vi "実測定画面.vi"(4 "測定値MAX/MIN":string[][](table), 7 "実測設定項目配列_\nメインからの転記":T1[](array[typedef]) {"測定モード" items=["単発測定モード", "連続測定モード", "多点測定モード"]}, 11 "測定周期/ms_制御器":dbl) -> (8 "実測設定項目配列_\nゲージIOへ転記用":T1[](array[typedef]) {"測定モード" items=["単発測定モード", "連続測定モード", "多点測定モード"]}, 10 "実測設定項目配列_\n多点測定メイン転記用":T1[](array[typedef]) {"測定モード" items=["単発測定モード", "連続測定モード", "多点測定モード"]}, 15 "測定周期/ms_表示器":dbl)   [LabVIEW 2021]
panel:
  out "文字列":string
  out "実測値MAXエラー判定 4":bool
  out "実測値MAXエラー判定 3":bool
  out "実測値MAXエラー判定 2":bool
  out "実測値MAXエラー判定":bool
  out "測定値MAX/MIN_グローバルから転記":string[][](table)
  in  "測定値MAX/MINリセット用 2":string[][](table)
  in  "測定値MAX/MIN_多点測定":string[][](table)
  in  "測定値MAX/MINリセット用":string[][](table)
  in  "実測ONOFFボタン":T2
  out "実測値":string[][](table)
  # "実測定画面"
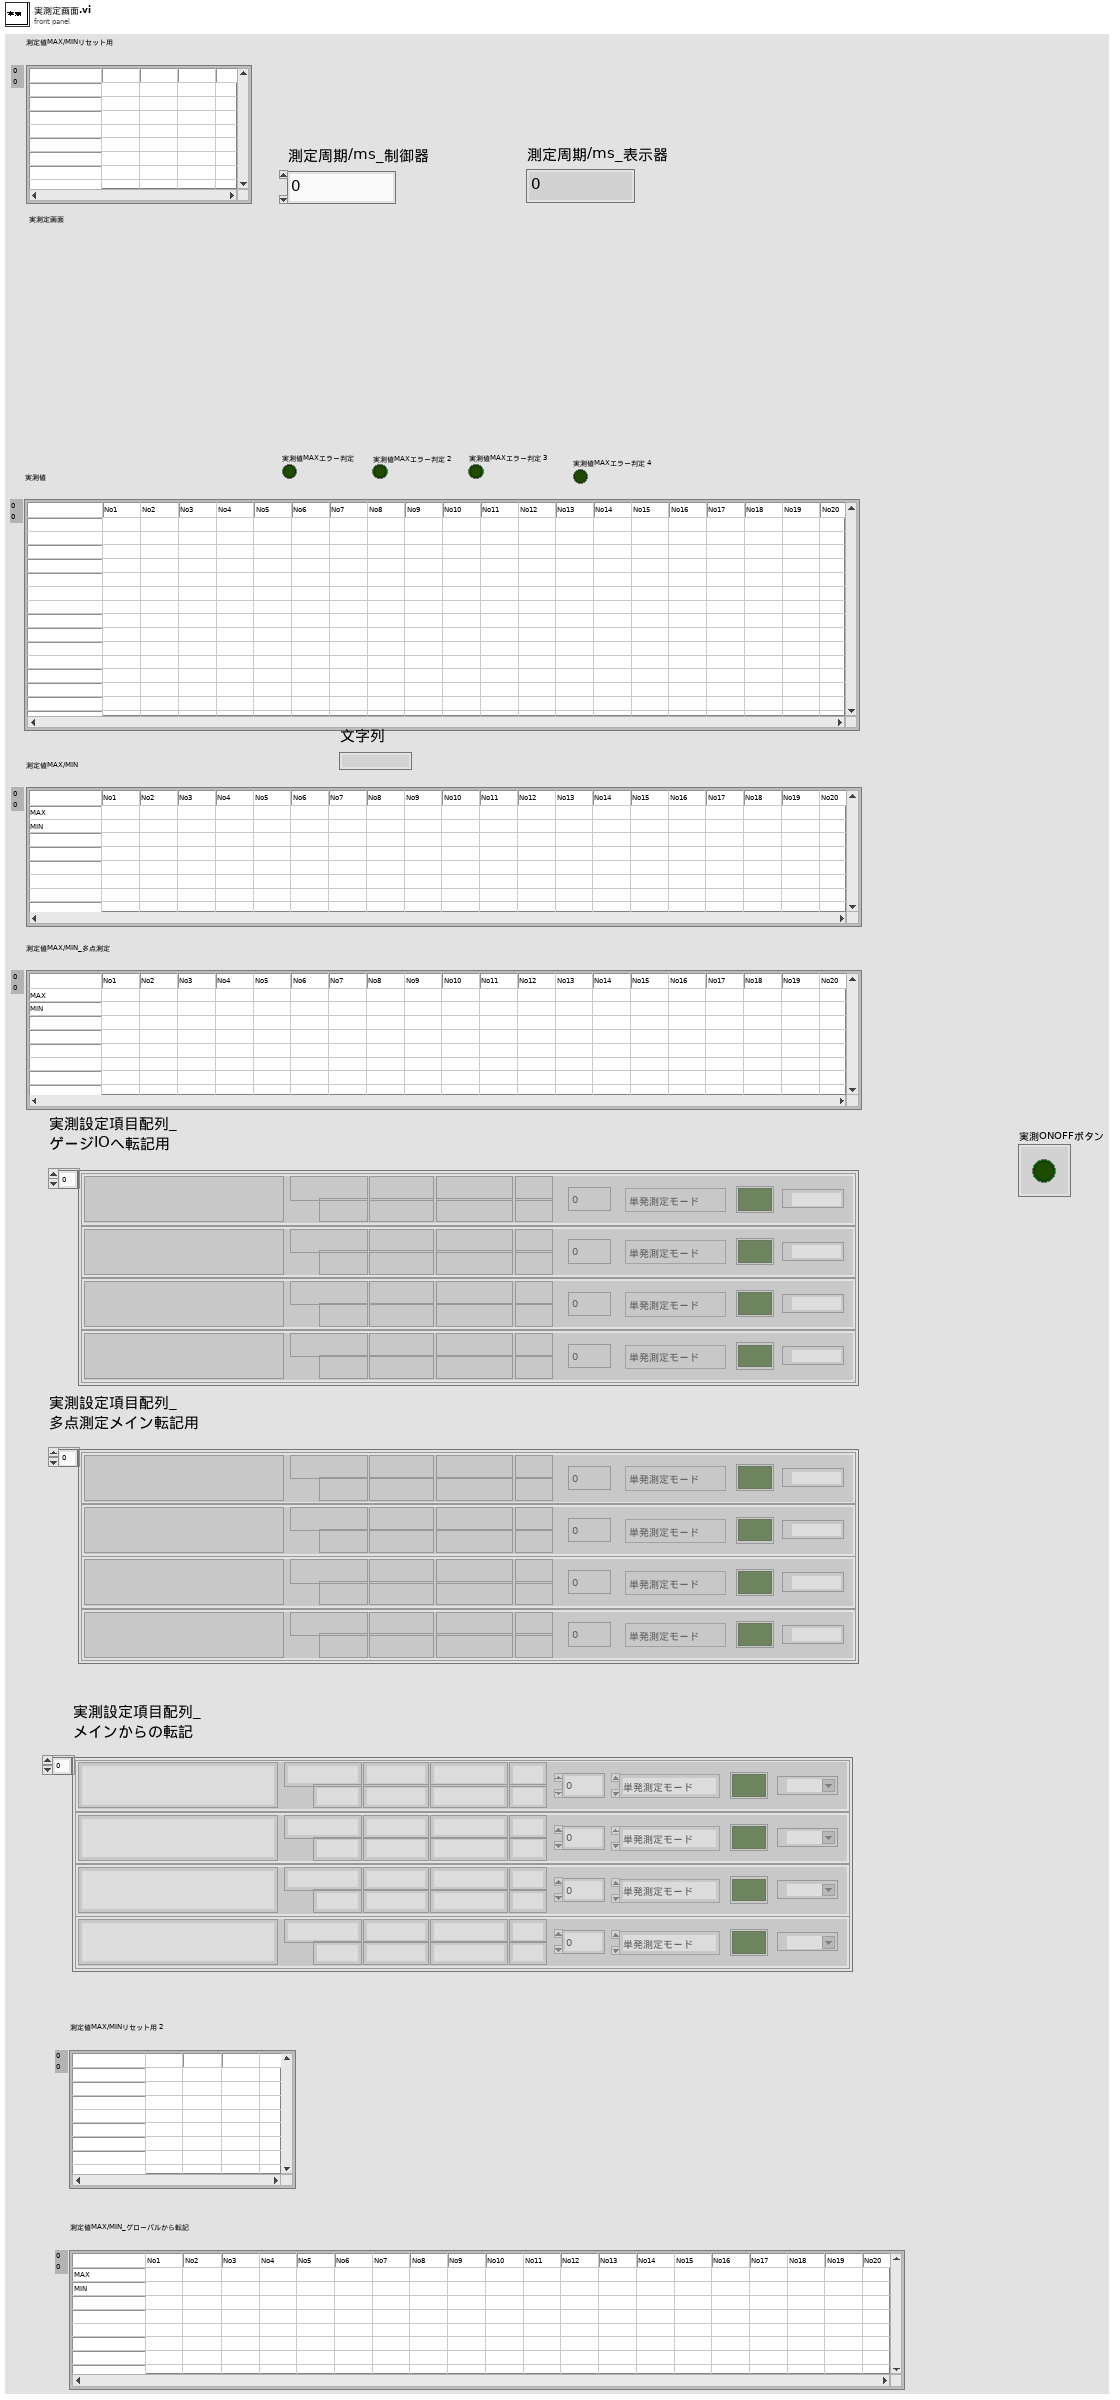
[diagram p1: front panel]
types:
  T1 = typedef "設定全項目制御器.ctl" = cluster{"規格":string, "規格上限":string, "規格下限":string, "ポートNo.":dbl, "測定モード":u16, "規格単位":string, "品質チェック項目":string, "測定周期":dbl, "実測値MAX":string, "実測値MIN":string, "実測値(MAX)":string, "実測値(MIN)":string, "測定画面表示ボタン":bool, "ゲージポートNo":refnum<visa-resource-name>}
  T2 = typedef "ONOFFボタン制御器.ctl" = cluster{"使用ON/OFF":bool}
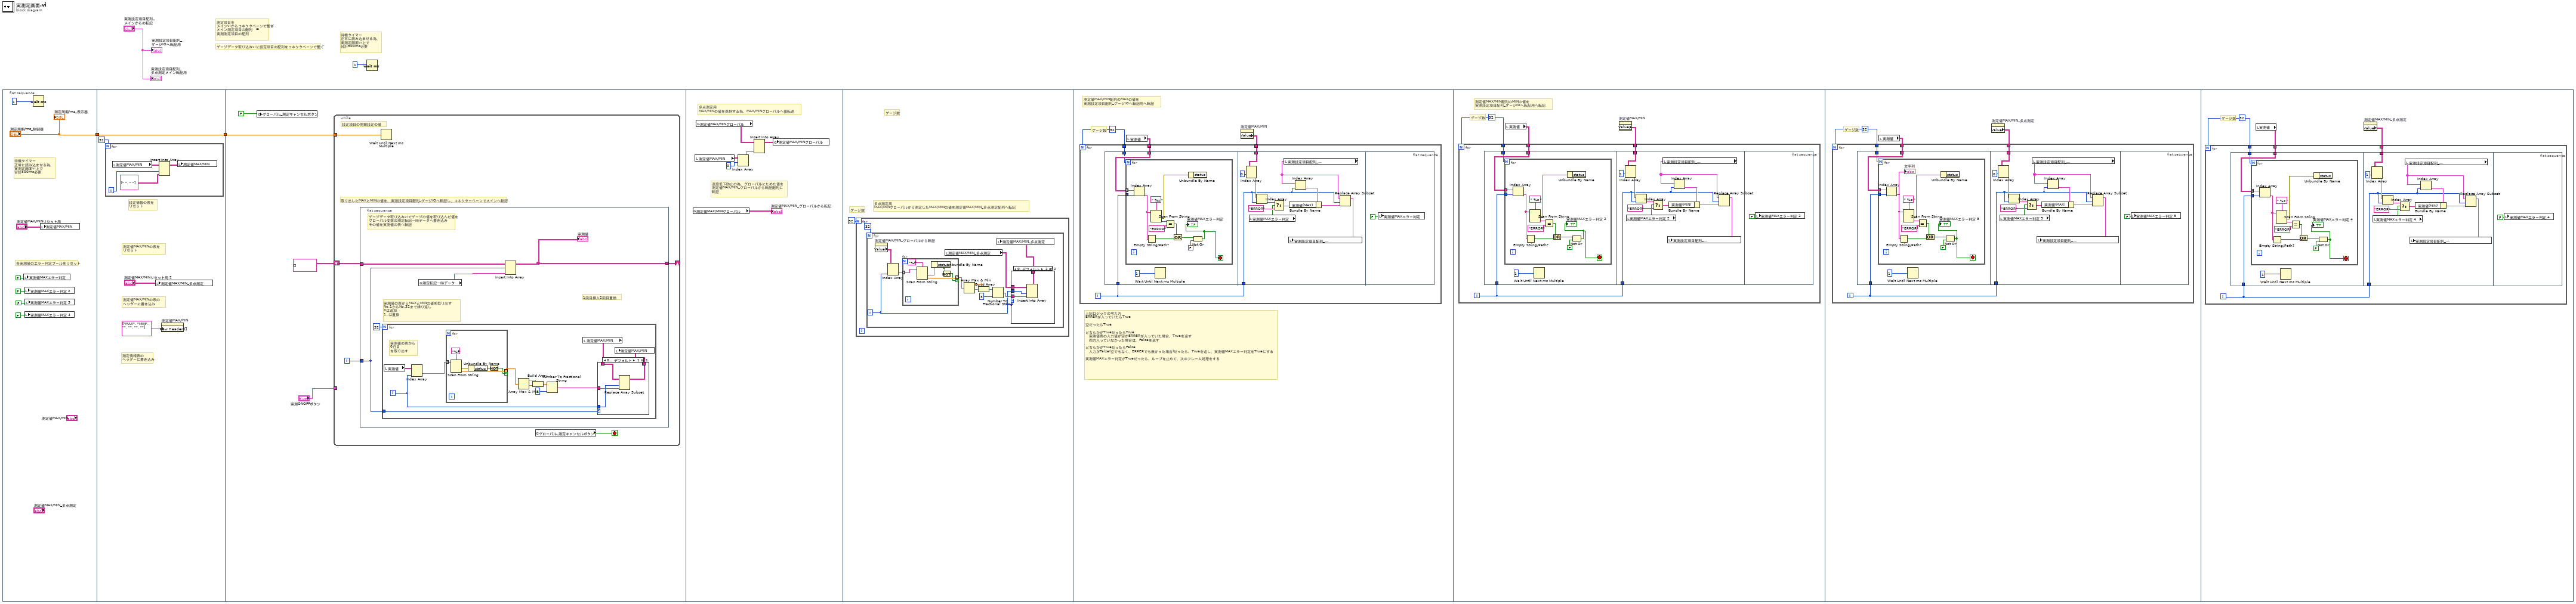
[diagram p0: block diagram]
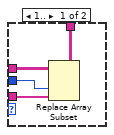
[diagram p2: hidden frame]
diagram:
  # "測定項目を\nメインviからコネクタペーンで繋ぎ\nメイン測定項目の配列　=\n実測測定項目の配列"
  # "ゲージデータ取り込みviに設定項目の配列をコネクタペーンで繋ぐ"
  # "待機タイマー\n正常に読み込ませる為、\n実測定画面vi上で\n合計500ms必要"
  n1 = flat-sequence {
    tunnel: ["測定周期/ms_制御器"] -> w4
    tunnel: w4 -> [w14]
    tunnel: [w14] -> w3
    tunnel: w3 -> [w21]
    frame #0 {
      # "各実測値のエラー判定ブールをリセット"
      # "待機タイマー\n正常に読み込ませる為、\n実測定画面vi上で\n合計500ms必要"
      n2 = local write "実測値MAXエラー判定"(FALSE) -> ()
      n3 = local write "実測値MAXエラー判定 2"(FALSE) -> ()
      n4 = local write "実測値MAXエラー判定 4"(FALSE) -> ()
      n5 = local write "実測値MAXエラー判定 3"(FALSE) -> ()
      n6 = Wait (ms)(milliseconds to wait=1) -> ()  [unwired: 1 out]
      n7 = local write "測定値MAX/MIN"("測定値MAX/MINリセット用") -> ()
      "測定周期/ms_表示器" <- "測定周期/ms_制御器"
    }
    frame #1 {
      # "測定情報表の\nヘッダーに書き込み"
      # "測定値MAX/MINの表の\nヘッダーに書き込み"
      # "測定値MAX/MINの表を\nリセット"
      # "設定情報の表を\nリセット"
      n8 = for {
        N: 32 -> [_]
        i -> [w16]
        n9 = local read "測定値MAX/MIN"() -> (w19:string[][])
        n10 = Insert Into Array(array=w19, index (col)=w16, new element=string[][] [[" "], [" "]]) -> (w18:string[][])  [unwired: 1 in]
        n11 = local write "測定値MAX/MIN"(w18) -> ()
      }
      n12 = local write "測定値MAX/MIN_多点測定"("測定値MAX/MINリセット用 2") -> ()
      n13 = property on="測定値MAX/MIN" class="Tbl (指定)"("Row Headers[]"=string[] ["MAX", "MIN", "", "", "", ""]) -> ()  [unwired: 2 in, 2 out]
    }
    frame #2 {
      n14 = global write "測定キャンセルボタン.vi" "グローバル_測定キャンセルボタン"(FALSE) -> ()
      n15 = while "Whileループ" {
        tunnel: "実測ONOFFボタン" -> [_]
        shift-right: [w26] -> _
        shift-left: string[][] [] ("配列") -> [w28]
        tunnel: w21 -> [w24]
        i -> [w27]
        stop <- w25 stop-if-true
        # "取り出したMAXとMINの値を、実測設定項目配列_ゲージIOへ転記し、コネクターペーンでメインへ転記"
        # "設定項目の周期設定の値"
        n16 = flat-sequence {
          tunnel: w28 -> [w33]
          tunnel: w27 -> [w29]
          tunnel: [w32] -> w26
          frame #0 {
            # "1回目挿入2回目置換"
            # "実測値の表からMAXとMINの値を取り出す\nNo.1からNo.32まで繰り返し\n0は追加\n1..は置換"
            # "ゲージデータ取り込みviでゲージの値を取り込んだ値を\nグローバル変数の測定転記一時データへ書き込み\nその値を実測値の表へ転記"
            n17 = for {
              N: 32 -> [_]
              tunnel: w29 -> [w41]
              i -> [w37]
              # "実測値の表から\n0行目\nを取り出す"
              n18 = local read "実測値"() -> (w45:string[][])
              n19 = Index Array(array=w45, index (col)=w37) -> (element=w34:string[])  [unwired: 1 in]
              n20 = for {
                tunnel: w34 -> [w54] mode=indexing
                tunnel: [w53] -> w42 mode=indexing if=w50
                n21 = Scan From String(format string="%f" ("形式文字列"), input string=w54) -> (error out=w52:errorcluster, output 1=w53:dbl)  [unwired: 3 in, 2 out]
                n22 = Unbundle By Name(w52) -> ("status"=w51:bool)
                n23 = Not(x=w51) -> (.not. x?=w50:bool)
              }
              n24 = Array Max & Min(array=w42) -> (max value=w36:dbl, min value=w44:dbl)  [unwired: 2 out]
              n25 = Build Array(w36, w44) -> (w43:dbl[])
              n26 = Number To Fractional String(number=w43, precision (6)=3) -> (F-format string=w35:string[])  [unwired: 2 in]
              n27 = local read "測定値MAX/MIN"() -> (w40:string[][])
              n28 = case shown="0.., デフォルト" w41 {
                tunnel: [w48] -> w39
                tunnel: w40 -> [w49]
                tunnel: w37 -> [w47]
                tunnel: w35 -> [w46]
                frame 0.., Default {
                  n29 = Replace Array Subset(array=w49, new element=w46, index (col)=w47) -> (w48:string[][])  [unwired: 1 in]
                }
              }
              n30 = local write "測定値MAX/MIN"(w39) -> ()
            }
            n31 = global read "測定データ転記.vi" "測定転記一時データ"() -> (w31:string[])
            n32 = Insert Into Array(array=w33, index (row)=w29, new element=w31) -> (w32:string[][])  [unwired: 1 in]
            "実測値" <- w32
          }
        }
        n33 = Wait Until Next ms Multiple(millisecond multiple=w24) -> ()  [unwired: 1 out]
        n34 = global read "測定キャンセルボタン.vi" "グローバル_測定キャンセルボタン"() -> (w25:bool)
      }
    }
    frame #3 {
      # "速度低下防止の為、グローバルにためた値を\n測定値MAX/MIN_グローバルから転記配列に\n転記"
      # "多点測定用\nMAX/MINの値を保持する為、MAX/MINグローバルへ値転送"
      n35 = global read "測定値MAXMIN_G.vi" "測定値MAX/MINグローバル"() -> (→"測定値MAX/MIN_グローバルから転記":string[][])
      n36 = local read "測定値MAX/MIN"() -> (w58:string[][])
      n37 = global read "測定値MAXMIN_G.vi" "測定値MAX/MINグローバル"() -> (w61:string[][])
      n38 = Index Array(array=w58, index (row)=0) -> (element=w59:string[])  [unwired: 1 in]
      n39 = Insert Into Array(array=w61, new element=w59) -> (w60:string[][])  [unwired: 2 in]
      n40 = global write "測定値MAXMIN_G.vi" "測定値MAX/MINグローバル"(w60) -> ()
    }
    frame #4 {
      # "多点測定用\nMAX/MINグローバルから測定したMAX/MINの値を測定値MAX/MIN_多点測定配列へ転記"
      # "ゲージ数"
      # "ゲージ数"
      n41 = for {
        N: 32 -> [_]
        n42 = for {
          N: 32 -> [_]
          i -> [w67]
          n43 = property on="測定値MAX/MIN_グローバルから転記" class="Tbl (指定)"() -> ("Value"=w65:string[][])  [unwired: 2 in, 2 out]
          n44 = Index Array(array=w65, index (col)=w67) -> (element=w71:string[])  [unwired: 1 in]
          n45 = for {
            tunnel: w71 -> [w88] mode=indexing
            tunnel: [w86] -> w70 mode=indexing if=w84
            n46 = Scan From String(format string="%f" ("形式文字列"), input string=w88) -> (error out=w85:errorcluster, output 1=w86:dbl)  [unwired: 3 in, 2 out]
            n47 = Unbundle By Name(w85) -> ("status"=w83:bool)
            n48 = Not(x=w83) -> (.not. x?=w84:bool)
          }
          n49 = local read "測定値MAX/MIN_多点測定"() -> (w69:string[][])
          n50 = Array Max & Min(array=w70) -> (max value=w74:dbl, min value=w66:dbl)  [unwired: 2 out]
          n51 = Build Array(w74, w66) -> (w73:dbl[])
          n52 = Number To Fractional String(number=w73, precision (6)=3) -> (F-format string=w72:string[])  [unwired: 2 in]
          n53 = case shown="0, デフォルト" w67 {
            tunnel: [w77 w80] -> w68
            tunnel: w69 -> [w78 w82]
            tunnel: w67 -> [w75 w79]
            tunnel: w72 -> [w76 w81]
            frame 1.. {
              n54 = Replace Array Subset(array=w78, new element=w76, index (col)=w75) -> (w77:string[][])  [unwired: 1 in]
            }
            frame 0, Default {
              n55 = Insert Into Array(array=w82, index (col)=w79, new element=w81) -> (w80:string[][])  [unwired: 1 in]
            }
          }
          n56 = local write "測定値MAX/MIN_多点測定"(w68) -> ()
        }
      }
    }
    frame #5 {
      w90 = 32
      # "上記ロジックの考え方\nERRERが入っていたらTrue\n\n空だったらTrue\n\nどちらかがTrueだったらTrue\n　実測値表の入力値が空かERRERが入っていた場合、Trueを返す\n　両方入っていなかった場合は、Falseを返す　\n\nどちらかがTrueだったらFalse\n　入力がFalse(空でもなく、ERRERでも無かった場合)だったら、Trueを返し、実測値MAXエラー判定をTrueにする\n\n実測値MAXエラー判定がTrueだったら、ループを止めて、次のフレーム処理をする"
      # "測定値MAX/MIN配列のMAXの値を\n実測設定項目配列_ゲージIOへ転記用へ転記"
      # "ゲージ数"
      n57 = local read "実測値"() -> (w91:string[][])
      n58 = property on="測定値MAX/MIN" class="Tbl (指定)"() -> ("Value"=w89:string[][])  [unwired: 2 in, 2 out]
      n59 = for {
        N: w90 -> [_]
        tunnel: w91 -> [w95]
        tunnel: w89 -> [w94]
        tunnel: w90 -> [w93]
        i -> [w92]
        n60 = flat-sequence {
          tunnel: w95 -> [w98]
          tunnel: w93 -> [w97]
          tunnel: w92 -> [w96]
          tunnel: w94 -> [w113]
          tunnel: w92 -> [w112]
          frame #0 {
            n61 = for {
              N: w97 -> [_]
              tunnel: w98 -> [w104] mode=indexing
              tunnel: w96 -> [w101]
              stop <- w100 stop-if-true
              n62 = Index Array(array=w104, index=w101) -> (element=w103:string)
              n63 = Empty String/Path?(string/path=w103) -> (empty?=w102:bool)
              n64 = Scan From String(format string=" %s " ("形式文字列"), input string=w103) -> (error out=w110:errorcluster, output 1=w109:string)  [unwired: 3 in, 2 out]
              n65 = Equal?(x=w109, y="ERROR") -> (x = y?=w107:bool)
              n66 = Or(x=w107, y=w102) -> (x .or. y?=w105:bool)
              n67 = Unbundle By Name(w110) -> ()  [unwired: 1 out]
              n68 = Not Or(1:FALSE, 2:w105) -> (0:w100:bool)
              "実測値MAXエラー判定" <- w100
            }
            n69 = Wait Until Next ms Multiple(millisecond multiple=u32 1 ("ミリ秒倍数")) -> ()  [unwired: 1 out]
          }
          frame #1 {
            n70 = Index Array(array=w113, index (row)=0) -> (element=w119:string[])  [unwired: 1 in]
            n71 = local read "実測値MAXエラー判定"() -> (w120:bool)
            n72 = Index Array(array=w119, index=w112) -> (element=w123:string)
            n73 = Select(t=w123, s=w120, f="ERROR") -> (s? t:f=w121:string)
            n74 = local read "実測設定項目配列_\nゲージIOへ転記用"() -> (w117:T1[])
            n75 = Index Array(array=w117, index=w112) -> (element=w114:T1)
            n76 = Bundle By Name(cluster=w114, "実測値(MAX)"=w121) -> (w115:T1)
            n77 = Replace Array Subset(array=w117, new element=w115, index=w112) -> (w116:T1[])
            n78 = local write "実測設定項目配列_\nゲージIOへ転記用"(w116) -> ()
          }
          frame #2 {
            n79 = local write "実測値MAXエラー判定"(FALSE) -> ()
          }
        }
      }
    }
    frame #6 {
      w127 = 32
      # "ゲージ数"
      # "測定値MAX/MIN配列のMINの値を\n実測設定項目配列_ゲージIOへ転記用へ転記"
      n80 = local read "実測値"() -> (w126:string[][])
      n81 = property on="測定値MAX/MIN" class="Tbl (指定)"() -> ("Value"=w125:string[][])  [unwired: 2 in, 2 out]
      n82 = for {
        N: w127 -> [_]
        tunnel: w126 -> [w131]
        tunnel: w125 -> [w130]
        tunnel: w127 -> [w129]
        i -> [w128]
        n83 = flat-sequence {
          tunnel: w131 -> [w134]
          tunnel: w129 -> [w133]
          tunnel: w128 -> [w132]
          tunnel: w130 -> [w149]
          tunnel: w128 -> [w148]
          frame #0 {
            n84 = for {
              N: w133 -> [_]
              tunnel: w134 -> [w140] mode=indexing
              tunnel: w132 -> [w137]
              stop <- w136 stop-if-true
              n85 = Index Array(array=w140, index=w137) -> (element=w139:string)
              n86 = Empty String/Path?(string/path=w139) -> (empty?=w138:bool)
              n87 = Scan From String(format string=" %s " ("形式文字列"), input string=w139) -> (error out=w146:errorcluster, output 1=w145:string)  [unwired: 3 in, 2 out]
              n88 = Equal?(x=w145, y="ERROR") -> (x = y?=w143:bool)
              n89 = Or(x=w143, y=w138) -> (x .or. y?=w141:bool)
              n90 = Unbundle By Name(w146) -> ()  [unwired: 1 out]
              n91 = Not Or(1:FALSE, 2:w141) -> (0:w136:bool)
              "実測値MAXエラー判定 2" <- w136
            }
            n92 = Wait Until Next ms Multiple(millisecond multiple=u32 1 ("ミリ秒倍数")) -> ()  [unwired: 1 out]
          }
          frame #1 {
            n93 = Index Array(array=w149, index (row)=1) -> (element=w155:string[])  [unwired: 1 in]
            n94 = local read "実測値MAXエラー判定 2"() -> (w156:bool)
            n95 = Index Array(array=w155, index=w148) -> (element=w159:string)
            n96 = Select(t=w159, s=w156, f="ERROR") -> (s? t:f=w157:string)
            n97 = local read "実測設定項目配列_\nゲージIOへ転記用"() -> (w153:T1[])
            n98 = Index Array(array=w153, index=w148) -> (element=w150:T1)
            n99 = Bundle By Name(cluster=w150, "実測値(MIN)"=w157) -> (w151:T1)
            n100 = Replace Array Subset(array=w153, new element=w151, index=w148) -> (w152:T1[])
            n101 = local write "実測設定項目配列_\nゲージIOへ転記用"(w152) -> ()
          }
          frame #2 {
            n102 = local write "実測値MAXエラー判定 2"(FALSE) -> ()
          }
        }
      }
    }
    frame #7 {
      w163 = 32
      # "ゲージ数"
      n103 = local read "実測値"() -> (w162:string[][])
      n104 = property on="測定値MAX/MIN_多点測定" class="Tbl (指定)"() -> ("Value"=w161:string[][])  [unwired: 2 in, 2 out]
      n105 = for {
        N: w163 -> [_]
        tunnel: w162 -> [w167]
        tunnel: w161 -> [w166]
        tunnel: w163 -> [w165]
        i -> [w164]
        n106 = flat-sequence {
          tunnel: w167 -> [w170]
          tunnel: w165 -> [w169]
          tunnel: w164 -> [w168]
          tunnel: w166 -> [w185]
          tunnel: w164 -> [w184]
          frame #0 {
            n107 = for {
              N: w169 -> [_]
              tunnel: w170 -> [w176] mode=indexing
              tunnel: w168 -> [w174]
              stop <- w172 stop-if-true
              n108 = Index Array(array=w176, index=w174) -> (element=w173:string)
              "文字列" <- w173
              n109 = Empty String/Path?(string/path=w173) -> (empty?=w175:bool)
              n110 = Scan From String(format string=" %s " ("形式文字列"), input string=w173) -> (error out=w182:errorcluster, output 1=w181:string)  [unwired: 3 in, 2 out]
              n111 = Equal?(x=w181, y="ERROR") -> (x = y?=w179:bool)
              n112 = Or(x=w179, y=w175) -> (x .or. y?=w177:bool)
              n113 = Unbundle By Name(w182) -> ()  [unwired: 1 out]
              n114 = Not Or(1:FALSE, 2:w177) -> (0:w172:bool)
              "実測値MAXエラー判定 3" <- w172
            }
            n115 = Wait Until Next ms Multiple(millisecond multiple=u32 1 ("ミリ秒倍数")) -> ()  [unwired: 1 out]
          }
          frame #1 {
            n116 = Index Array(array=w185, index (row)=0) -> (element=w191:string[])  [unwired: 1 in]
            n117 = local read "実測値MAXエラー判定 3"() -> (w192:bool)
            n118 = Index Array(array=w191, index=w184) -> (element=w195:string)
            n119 = Select(t=w195, s=w192, f="ERROR") -> (s? t:f=w193:string)
            n120 = local read "実測設定項目配列_\n多点測定メイン転記用"() -> (w189:T1[])
            n121 = Index Array(array=w189, index=w184) -> (element=w186:T1)
            n122 = Bundle By Name(cluster=w186, "実測値(MAX)"=w193) -> (w187:T1)
            n123 = Replace Array Subset(array=w189, new element=w187, index=w184) -> (w188:T1[])
            n124 = local write "実測設定項目配列_\n多点測定メイン転記用"(w188) -> ()
          }
          frame #2 {
            n125 = local write "実測値MAXエラー判定 3"(FALSE) -> ()
          }
        }
      }
    }
    frame #8 {
      w198 = 32
      # "ゲージ数"
      n126 = local read "実測値"() -> (w199:string[][])
      n127 = property on="測定値MAX/MIN_多点測定" class="Tbl (指定)"() -> ("Value"=w197:string[][])  [unwired: 2 in, 2 out]
      n128 = for {
        N: w198 -> [_]
        tunnel: w199 -> [w203]
        tunnel: w197 -> [w202]
        tunnel: w198 -> [w201]
        i -> [w200]
        n129 = flat-sequence {
          tunnel: w203 -> [w206]
          tunnel: w201 -> [w205]
          tunnel: w200 -> [w204]
          tunnel: w202 -> [w221]
          tunnel: w200 -> [w220]
          frame #0 {
            n130 = for {
              N: w205 -> [_]
              tunnel: w206 -> [w212] mode=indexing
              tunnel: w204 -> [w209]
              stop <- w208 stop-if-true
              n131 = Index Array(array=w212, index=w209) -> (element=w211:string)
              n132 = Empty String/Path?(string/path=w211) -> (empty?=w210:bool)
              n133 = Scan From String(format string=" %s " ("形式文字列"), input string=w211) -> (error out=w218:errorcluster, output 1=w217:string)  [unwired: 3 in, 2 out]
              n134 = Equal?(x=w217, y="ERROR") -> (x = y?=w215:bool)
              n135 = Or(x=w215, y=w210) -> (x .or. y?=w213:bool)
              n136 = Unbundle By Name(w218) -> ()  [unwired: 1 out]
              n137 = Not Or(1:FALSE, 2:w213) -> (0:w208:bool)
              "実測値MAXエラー判定 4" <- w208
            }
            n138 = Wait Until Next ms Multiple(millisecond multiple=u32 1 ("ミリ秒倍数")) -> ()  [unwired: 1 out]
          }
          frame #1 {
            n139 = Index Array(array=w221, index (row)=1) -> (element=w227:string[])  [unwired: 1 in]
            n140 = local read "実測値MAXエラー判定 4"() -> (w228:bool)
            n141 = Index Array(array=w227, index=w220) -> (element=w231:string)
            n142 = Select(t=w231, s=w228, f="ERROR") -> (s? t:f=w229:string)
            n143 = local read "実測設定項目配列_\n多点測定メイン転記用"() -> (w225:T1[])
            n144 = Index Array(array=w225, index=w220) -> (element=w222:T1)
            n145 = Bundle By Name(cluster=w222, "実測値(MIN)"=w229) -> (w223:T1)
            n146 = Replace Array Subset(array=w225, new element=w223, index=w220) -> (w224:T1[])
            n147 = local write "実測設定項目配列_\n多点測定メイン転記用"(w224) -> ()
          }
          frame #2 {
            n148 = local write "実測値MAXエラー判定 4"(FALSE) -> ()
          }
        }
      }
    }
  }
  n149 = Wait (ms)(milliseconds to wait=1) -> ()  [unwired: 1 out]
  "実測設定項目配列_\nゲージIOへ転記用" <- "実測設定項目配列_\nメインからの転記"
  "実測設定項目配列_\n多点測定メイン転記用" <- "実測設定項目配列_\nメインからの転記"
